vi "AutoSequencer.vi"(2 "Reinit Sequencer":bool, 7 "Auto Cluster In":T1) -> (8 "Auto Cluster Out":T1)   [LabVIEW 2023]
doc: "This VI manages the autonomous sequence. The drive base and manipulator sequencers operate in parallel. Autonomous plays are written as text files and uploaded to the roboRIO via FileZilla. The appropriate play is slected prior to the match via the FRC 4265 Dashboard. For each sequencer, each step is composed of a command and a parameter string of arbitrary length. Error checking and handling is supported. An autonomous test mode (for simulating autonomous plays on the robot cart) is supported. Status updates are sent to the FRC Driver Station and the FRC 4265 Dashboard throughout autonomous. Note that the autonomous sequencer may be also active during the begining of TeleOperated mode, as determined by the MasterRobotModeController.vi."
uses:
  GlobalPoseAndTargeting.vi
  GlobalDriverStationData.vi
  GlobalAutonomous.vi
panel:
  in  "Type Def":T1
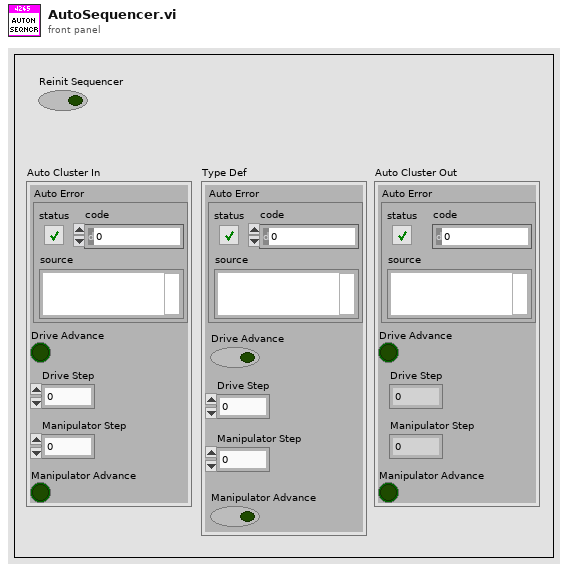
[diagram p1: front panel]
types:
  T1 = cluster{"Auto Error":errorcluster, "Drive Advance":bool, "Drive Step":i32, "Manipulator Step":i32, "Manipulator Advance":bool}
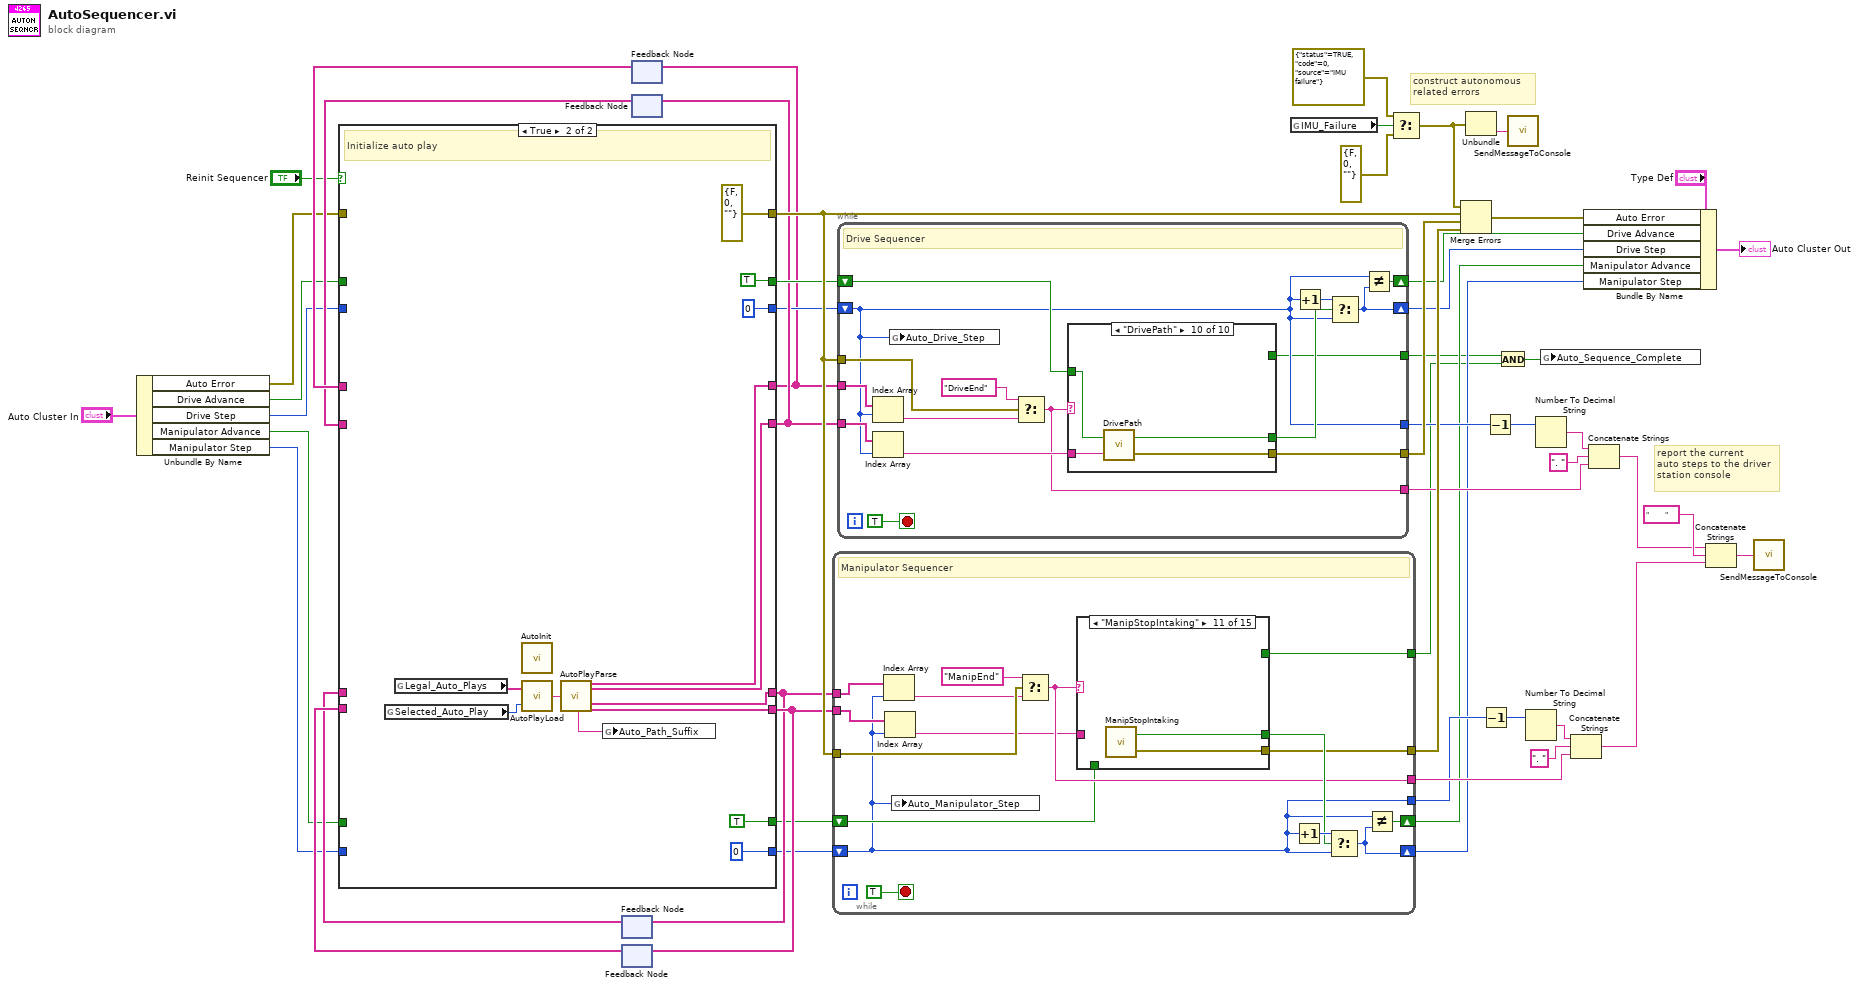
[diagram p0: block diagram]
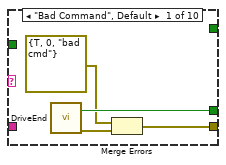
[diagram p2: hidden frame]
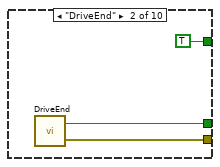
[diagram p3: hidden frame]
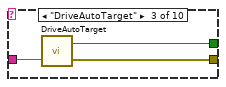
[diagram p4: hidden frame]
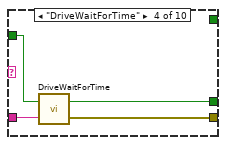
[diagram p5: hidden frame]
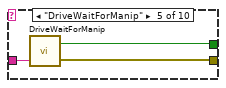
[diagram p6: hidden frame]
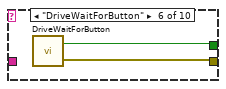
[diagram p7: hidden frame]
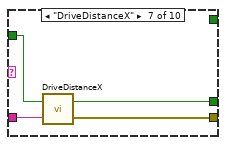
[diagram p8: hidden frame]
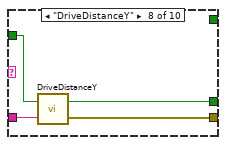
[diagram p9: hidden frame]
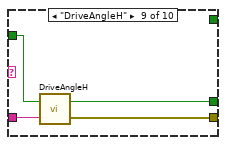
[diagram p10: hidden frame]
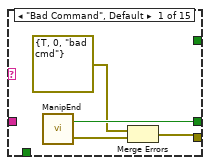
[diagram p12: hidden frame]
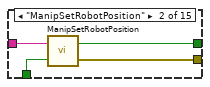
[diagram p13: hidden frame]
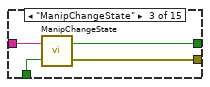
[diagram p14: hidden frame]
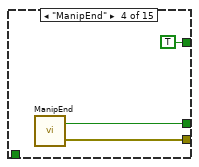
[diagram p15: hidden frame]
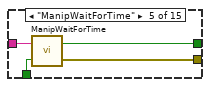
[diagram p16: hidden frame]
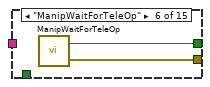
[diagram p17: hidden frame]
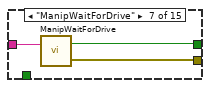
[diagram p18: hidden frame]
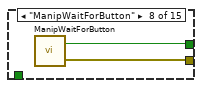
[diagram p19: hidden frame]
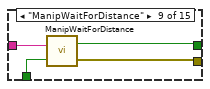
[diagram p20: hidden frame]
diagram:
  # "construct autonomous\nrelated errors"
  # "report the current\nauto steps to the driver\nstation console"
  n1 = Unbundle By Name("Auto Cluster In") -> ("Auto Error"=w12:errorcluster, "Drive Advance"=w11:bool, "Drive Step"=w10:i32, "Manipulator Advance"=w9:bool, "Manipulator Step"=w8:i32)
  n2 = feedback #1() -> (w42:string[])  [unwired: 1 in]
  n3 = feedback #2() -> (w43:string[])  [unwired: 1 in]
  n4 = feedback #3() -> (w47:string[])  [unwired: 1 in]
  n5 = feedback #4() -> (w46:string[])  [unwired: 1 in]
  n6 = case shown="True" "Reinit Sequencer" {
    tunnel: w8 -> [w59 _]
    tunnel: w9 -> [w60 _]
    tunnel: [w60 TRUE ("Advance Trigger")] -> w29
    tunnel: [w59 0] -> w38
    tunnel: [w58 w67] -> w40
    tunnel: [w57 w71] -> w41
    tunnel: w42 -> [w58 _]
    tunnel: w43 -> [w57 _]
    tunnel: [w56 0] -> w44
    tunnel: w10 -> [w56 _]
    tunnel: [w55 w69] -> w45
    tunnel: [w54 w68] -> w1
    tunnel: w46 -> [w55 _]
    tunnel: w47 -> [w54 _]
    tunnel: [w53 TRUE] -> w48
    tunnel: w11 -> [w53 _]
    tunnel: [w52 errorcluster {"status"=FALSE, "code"=0, "source"=""} ("error constant")] -> w50
    tunnel: w12 -> [w52 _]
    frame False {
      # "Continue auto play"
    }
    frame True {
      # "Initialize auto play"
      n7 = global read "GlobalDriverStationData.vi" "Selected_Auto_Play"() -> (w65:u16)
      n8 = global read "GlobalAutonomous.vi" "Legal_Auto_Plays"() -> (w63:string[])
      n9 = call "AutoInit.vi"() -> ()  [unwired: 1 in]
      n10 = call "AutoPlayLoad.vi"("Selected Auto Play"=w65, "Available Auto Plays"=w63) -> ("Loaded Auto Play"=w62:string)
      n11 = call "AutoPlayParse.vi"("Loaded Auto Play"=w62) -> ("Autonomous Path Suffix"=w61:string, "Drive Command Strings"=w68:string[], "Drive Parameter Strings"=w69:string[], "Manipulator Command Strings"=w67:string[], "Manipulator Parameter Strings"=w71:string[])  [unwired: 10 in, 4 out]
      n12 = global write "GlobalAutonomous.vi" "Auto_Path_Suffix"(w61) -> ()
    }
  }
  n13 = feedback-in #1(w40) -> ()
  n14 = feedback-in #2(w41) -> ()
  n15 = feedback-in #3(w1) -> ()
  n16 = feedback-in #4(w45) -> ()
  n17 = while {
    tunnel: w40 -> [w85]
    shift-right: [w87] -> w15
    shift-left: w38 -> [w75]
    shift-right: [w86] -> w16
    shift-left: w29 -> [w77]
    tunnel: w41 -> [w84]
    tunnel: [w79] -> w32
    tunnel: [w80] -> w51
    tunnel: w50 -> [w82]
    tunnel: [w75] -> w23
    tunnel: [w74] -> w5
    stop <- TRUE stop-if-true
    # "Manipulator Sequencer"
    n18 = Index Array(array=w85, index=w75) -> (element=w76:string)
    n19 = Index Array(array=w84, index=w75) -> (element=w78:string)
    n20 = global write "GlobalAutonomous.vi" "Auto_Manipulator_Step"(w75) -> ()
    n21 = Select(t="ManipEnd", s=w82, f=w76) -> (s? t:f=w79:string)
    n22 = case shown="\"ManipStopIntaking\"" w79 {
      tunnel: w78 -> [_ w94 w101 _ w108 _ w113 _ w119 w123 _ w128 _ w133 w136]
      tunnel: [w93 w97 w100 w104 w106 w110 w112 w115 w117 w122 w125 w127 w130 w131 w134] -> w81
      tunnel: [w91 w96 w99 w103 w105 w109 w111 w114 w116 w121 w124 w126 w129 w132 w135] -> w80
      tunnel: w77 -> [_ w95 w98 _ w107 _ _ _ w118 w120 _ _ _ _ _]
      tunnel: [_ _ _ TRUE _ _ _ _ _ _ _ _ _ _ _] -> w74
      frame "Bad Command", Default {
        n23 = call "ManipEnd.vi"() -> ("Error Out"=w92:errorcluster, "Advance Trigger"=w93:bool)  [unwired: 2 in]
        n24 = Merge Errors(errorcluster {"status"=TRUE, "code"=0, "source"="bad cmd"} ("Path Follow Error"), w92) -> (w91:errorcluster)
      }
      frame "ManipSetRobotPosition" {
        n25 = call "ManipSetRobotPosition.vi"("Reinit"=w95, "Parameter String"=w94) -> ("Error Out"=w96:errorcluster, "Advance Trigger"=w97:bool)
      }
      frame "ManipChangeState" {
        n26 = call "ManipChangeState.vi"("Reinit"=w98, "Instruction String"=w101) -> ("Error Out"=w99:errorcluster, "Advance Trigger"=w100:bool)
      }
      frame "ManipEnd" {
        n27 = call "ManipEnd.vi"() -> ("Error Out"=w103:errorcluster, "Advance Trigger"=w104:bool)  [unwired: 2 in]
      }
      frame "ManipWaitForTime" {
        n28 = call "ManipWaitForTime.vi"("Reinit"=w107, "Parameter String"=w108) -> ("Error Out"=w105:errorcluster, "Advance Trigger"=w106:bool)
      }
      frame "ManipWaitForTeleOp" {
        n29 = call "ManipWaitForTeleOp.vi"() -> ("Error Out"=w109:errorcluster, "Advance Trigger"=w110:bool)  [unwired: 2 in]
      }
      frame "ManipWaitForDrive" {
        n30 = call "ManipWaitForDrive.vi"("Parameter String"=w113) -> ("Error Out"=w111:errorcluster, "Advance Trigger"=w112:bool)  [unwired: 1 in]
      }
      frame "ManipWaitForButton" {
        n31 = call "ManipWaitForButton.vi"() -> ("Error Out"=w114:errorcluster, "Advance Trigger"=w115:bool)  [unwired: 2 in]
      }
      frame "ManipWaitForDistance" {
        n32 = call "ManipWaitForDistance.vi"("Reinit"=w118, "Parameter String"=w119) -> ("Error Out"=w116:errorcluster, "Advance Trigger"=w117:bool)
      }
      frame "ManipSetIntaking" {
        n33 = call "ManipSetIntaking.vi"("Reinit"=w120, "Parameter String"=w123) -> ("Error Out"=w121:errorcluster, "Advance Trigger"=w122:bool)
      }
      frame "ManipStopIntaking" {
        n34 = call "ManipStopIntaking.vi"() -> ("Error Out"=w124:errorcluster, "Advance Trigger"=w125:bool)  [unwired: 2 in]
      }
      frame "ManipSetShooting" {
        n35 = call "ManipSetShooting.vi"("Parameter String"=w128) -> ("Error Out"=w126:errorcluster, "Advance Trigger"=w127:bool)  [unwired: 1 in]
      }
      frame "ManipWaitForPiece" {
        n36 = call "ManipWaitForPiece.vi"() -> ("Error Out"=w129:errorcluster, "Advance Trigger"=w130:bool)  [unwired: 2 in]
      }
      frame "ManipShooterPrespin" {
        n37 = call "ManipShooterPrespin.vi"("Parameter String"=w133) -> ("Error Out"=w132:errorcluster, "Advance Trigger"=w131:bool)  [unwired: 1 in]
      }
      frame "ManipReverseIntake" {
        n38 = call "ManipReverseIntake.vi"("Parameter String"=w136) -> ("Error Out"=w135:errorcluster, "Advance Trigger"=w134:bool)  [unwired: 1 in]
      }
    }
    n39 = Increment(x=w75) -> (x+1=w89:i32)
    n40 = Select(t=w89, s=w81, f=w75) -> (s? t:f=w87:i32)
    n41 = Not Equal?(x=w75, y=w87) -> (x != y?=w86:bool)
  }
  n42 = while {
    shift-right: [w147] -> w17
    shift-left: w44 -> [w138]
    tunnel: w1 -> [w150]
    tunnel: w45 -> [w149]
    shift-right: [w146] -> w18
    shift-left: w48 -> [w145]
    tunnel: [w139] -> w37
    tunnel: w50 -> [w143]
    tunnel: [w140] -> w49
    tunnel: [w138] -> w24
    tunnel: [w137] -> w6
    stop <- TRUE stop-if-true
    # "Drive Sequencer"
    n43 = Index Array(array=w150, index=w138) -> (element=w142:string)
    n44 = Index Array(array=w149, index=w138) -> (element=w148:string)
    n45 = global write "GlobalAutonomous.vi" "Auto_Drive_Step"(w138) -> ()
    n46 = Select(t="DriveEnd", s=w143, f=w142) -> (s? t:f=w139:string)
    n47 = case shown="\"DrivePath\"" w139 {
      tunnel: w148 -> [_ _ w160 w164 w169 _ w174 w177 w181 w186]
      tunnel: [w156 w159 w162 w165 w167 w171 w173 w179 w183 w184] -> w144
      tunnel: w145 -> [_ _ _ w163 _ _ w175 w178 w182 w187]
      tunnel: [w154 w158 w161 w166 w168 w170 w172 w176 w180 w185] -> w140
      tunnel: [_ TRUE _ _ _ _ _ _ _ _] -> w137
      frame "Bad Command", Default {
        n48 = call "DriveEnd.vi"() -> ("Error Out"=w155:errorcluster, "Advance Trigger"=w156:bool)  [unwired: 2 in]
        n49 = Merge Errors(errorcluster {"status"=TRUE, "code"=0, "source"="bad cmd"} ("Path Follow Error"), w155) -> (w154:errorcluster)
      }
      frame "DriveEnd" {
        n50 = call "DriveEnd.vi"() -> ("Error Out"=w158:errorcluster, "Advance Trigger"=w159:bool)  [unwired: 2 in]
      }
      frame "DriveAutoTarget" {
        n51 = call "DriveAutoTarget.vi"("Parameter String"=w160) -> ("Error Out"=w161:errorcluster, "Increment"=w162:bool)  [unwired: 1 in]
      }
      frame "DriveWaitForTime" {
        n52 = call "DriveWaitForTime.vi"("Parameter String"=w164, "Reinit"=w163) -> ("Error Out"=w166:errorcluster, "Increment"=w165:bool)
      }
      frame "DriveWaitForManip" {
        n53 = call "DriveWaitForManip.vi"("Parameter String"=w169) -> ("Error Out"=w168:errorcluster, "Increment"=w167:bool)  [unwired: 1 in]
      }
      frame "DriveWaitForButton" {
        n54 = call "DriveWaitForButton.vi"() -> ("Error Out"=w170:errorcluster, "Increment"=w171:bool)  [unwired: 2 in]
      }
      frame "DriveDistanceX" {
        n55 = call "DriveDistanceX.vi"("Parameter String"=w174, "Reinit"=w175) -> ("Error Out"=w172:errorcluster, "Increment"=w173:bool)
      }
      frame "DriveDistanceY" {
        n56 = call "DriveDistanceY.vi"("Parameter String"=w177, "Reinit"=w178) -> ("Error Out"=w176:errorcluster, "Increment"=w179:bool)
      }
      frame "DriveAngleH" {
        n57 = call "DriveAngleH.vi"("Parameter String"=w181, "Reinit"=w182) -> ("Error Out"=w180:errorcluster, "Increment"=w183:bool)
      }
      frame "DrivePath" {
        n58 = call "DrivePath.vi"("Parameter String"=w186, "Reinit"=w187) -> ("Path Follower Error"=w185:errorcluster, "Increment"=w184:bool)
      }
    }
    n59 = Increment(x=w138) -> (x+1=w151:i32)
    n60 = Select(t=w151, s=w144, f=w138) -> (s? t:f=w147:i32)
    n61 = Not Equal?(x=w138, y=w147) -> (x != y?=w146:bool)
  }
  n62 = global read "GlobalPoseAndTargeting.vi" "IMU_Failure"() -> (w20:bool)
  n63 = Select(t=errorcluster {"status"=TRUE, "code"=0, "source"="IMU failure"} ("error constant"), s=w20, f=errorcluster {"status"=FALSE, "code"=0, "source"=""} ("error constant")) -> (s? t:f=w22:errorcluster)
  n64 = Merge Errors(w22, w50, w49, w51) -> (w19:errorcluster)
  n65 = Unbundle(w22) -> ("source"=w21:string)  [unwired: 2 out]
  n66 = Decrement(x=w23) -> (x-1=w2:i32)
  n67 = Decrement(x=w24) -> (x-1=w3:i32)
  n68 = And(x=w6, y=w5) -> (x .and. y?=w7:bool)
  n69 = call "SendMessageToConsole.vi"("Message String"=w21) -> ()  [unwired: 1 in]
  n70 = Number To Decimal String(number=w2) -> (decimal integer string=w33:string)  [unwired: 1 in]
  n71 = Number To Decimal String(number=w3) -> (decimal integer string=w35:string)  [unwired: 1 in]
  n72 = global write "GlobalAutonomous.vi" "Auto_Sequence_Complete"(w7) -> ()
  n73 = Concatenate Strings(w33, ". " ("string"), w32) -> (w26:string)
  n74 = Bundle By Name(cluster="Type Def", "Auto Error"=w19, "Drive Advance"=w18, "Drive Step"=w17, "Manipulator Advance"=w16, "Manipulator Step"=w15) -> (→"Auto Cluster Out":T1)
  n75 = Concatenate Strings(w35, ". " ("string"), w37) -> (w27:string)
  n76 = Concatenate Strings(w27, "        " ("string"), w26) -> (w25:string)
  n77 = call "SendMessageToConsole.vi"("Message String"=w25) -> ()  [unwired: 1 in]
